vi "Read Fluid file_d.vi"(6 "error in (no error)":errorcluster, 9 "Fluid File":path) -> (0 "error out":errorcluster, 2 "Fluid Cluster":T1)   [LabVIEW 2017]
doc: "Reads the .mix file from the disk and retruns a cluster specifying the composition of the fluid.\n\nDeveloped by:\nGreg Sussman\nProcess Automation Corp\nwww.processauto.com\n(267)685-1249"
uses:
  Mixture Composition cluster_d.ctl
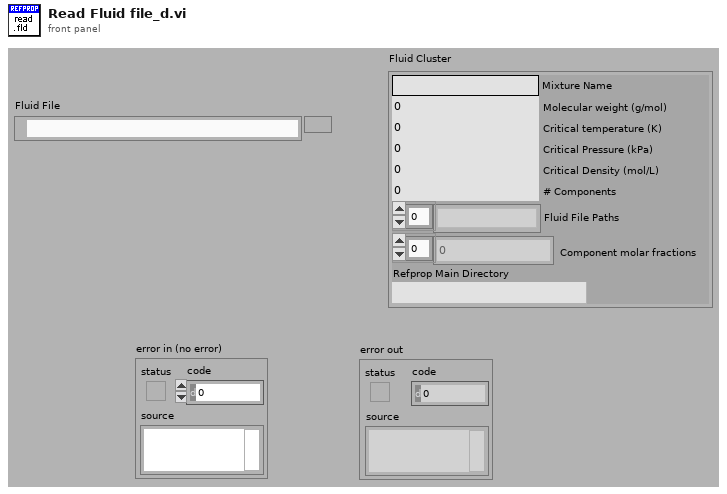
[diagram p1: front panel]
types:
  T1 = typedef "Mixture Composition cluster_d.ctl" = cluster{"Mixture Name":string, "Molecular weight (g/mol)":dbl, "Critical temperature (K)":dbl, "Critical Pressure (kPa)":dbl, "Critical Density (mol/L)":dbl, "# Components":i32, "Fluid File Paths":path[], "Component molar fractions":dbl[], "Refprop Main Directory":path}
  T2 = enum16{"open", "open or create", "create or replace", "create", "open (read only)"}
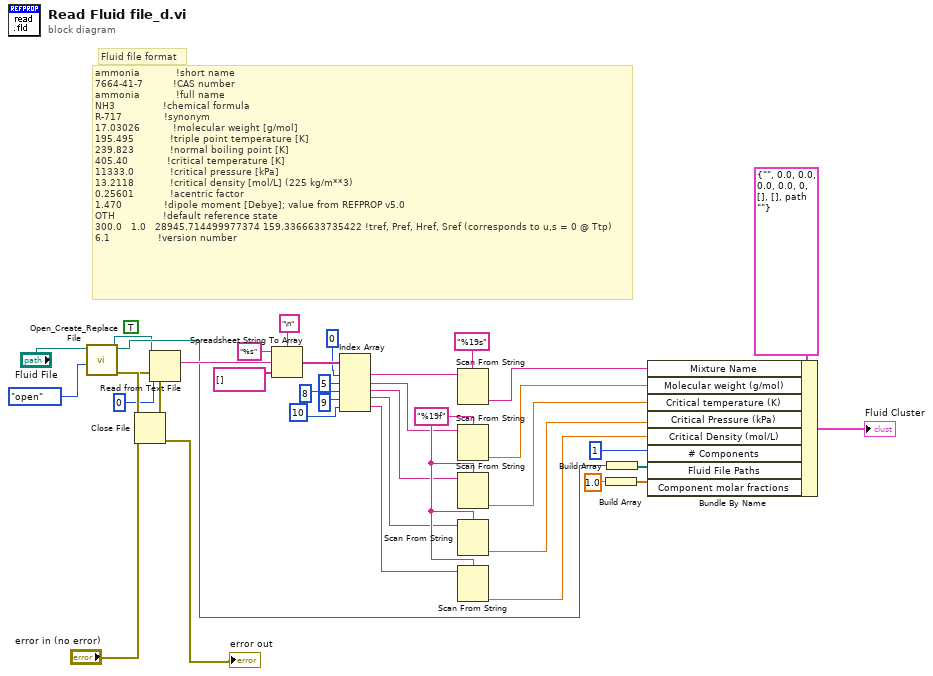
[diagram p0: block diagram]
diagram:
  (unwired) TRUE ("convert eol (F)")
  w17 = "%19f"
  # "Fluid file format"
  # "ammonia            !short name\n7664-41-7          !CAS number\nammonia            !full name\nNH3                !chemical formula\nR-717              !synonym\n17.03026           !molecular weight [g/mol]\n195.495            !triple point temperature [K]\n239.823            !normal boiling point [K]\n405.40             !critical temperature [K]\n11333.0            !critical pressure [kPa]\n13.2118            !critical density [mol/L] (225 kg/m**3)\n0.25601            !acentric factor\n1.470              !dipole moment [Debye]; value from REFPROP v5.0\nOTH                !default reference state\n300.0   1.0   28945.714499977374 159.3366633735422 !tref, Pref, Href, Sref (corresponds to u,s = 0 @ Ttp)\n6.1                !version number"
  n1 = call <vilib>:"Open_Create_Replace File.vi"("error in (no error)"="error in (no error)", "function (open:0)"=T2."open", "file path"="Fluid File") -> ("error out"=w6:errorcluster, "refnum"=w5:refnum<file>)  [unwired: 5 in, 2 out]
  n2 = Read from Text File(file (use dialog)=w5, count=0 ("计数"), error in=w6) -> (refnum out=w3:refnum<file>, text=w31:string, error out=w4:errorcluster)  [unwired: 1 in, 1 out]
  n3 = Close File(refnum=w3, error in=w4) -> (error out=→"error out":errorcluster)  [unwired: 1 out]
  n4 = Spreadsheet String To Array(delimiter (Tab)="\n", format string="%s", spreadsheet string=w31, array type (2D Dbl)=string[] []) -> (array=w34:string[])
  n5 = Index Array(array=w34, index #1=0, index #2=5 ("index"), index #3=8 ("index"), index #4=9 ("index"), index #5=10 ("index")) -> (element #1=w19:string, element #2=w12:string, element #3=w11:string, element #4=w10:string, element #5=w9:string)
  n6 = Scan From String(format string="%19s", input string=w19) -> (output 1=w18:string)  [unwired: 3 in, 3 out]
  n7 = Scan From String(format string=w17, input string=w12) -> (output 1=w16:dbl)  [unwired: 3 in, 3 out]
  n8 = Scan From String(format string=w17, input string=w11) -> (output 1=w15:dbl)  [unwired: 3 in, 3 out]
  n9 = Scan From String(format string=w17, input string=w10) -> (output 1=w14:dbl)  [unwired: 3 in, 3 out]
  n10 = Scan From String(format string=w17, input string=w9) -> (output 1=w13:dbl)  [unwired: 3 in, 3 out]
  n11 = Build Array(1.0) -> (w23:dbl[])
  n12 = Build Array("Fluid File") -> (w21:path[])
  n13 = Bundle By Name(cluster=T1 {"Mixture Name"="", "Molecular weight (g/mol)"=0.0, "Critical temperature (K)"=0.0, "Critical Pressure (kPa)"=0.0, "Critical Density (mol/L)"=0.0, "# Components"=0, "Fluid File Paths"=[], "Component molar fractions"=[], "Refprop Main Directory"=path ""} ("Mixure Cluster"), "Mixture Name"=w18, "Molecular weight (g/mol)"=w16, "Critical temperature (K)"=w15, "Critical Pressure (kPa)"=w14, "Critical Density (mol/L)"=w13, "# Components"=1, "Fluid File Paths"=w21, "Component molar fractions"=w23) -> (→"Fluid Cluster":T1)
